vi "项操作.vi"(8 "error in (no error)":errorcluster caption="错误输入（无错误）", 9 "Cell Position":T1, 10 "MCListbox引用句柄":refnum<vi>, 11 "LNK 输入":refnum<class "Hide Row.lvclass">) -> (0 "error out":errorcluster caption="错误输出", 3 "LNK 输出":refnum<class "Hide Row.lvclass">)   [LabVIEW 2016, in "Hide Row.lvclass"]
uses:
  Hide Row.lvclass
  <vilib>/Utility/miscctls.llb/LVRowAndColumnTypeDef.ctl
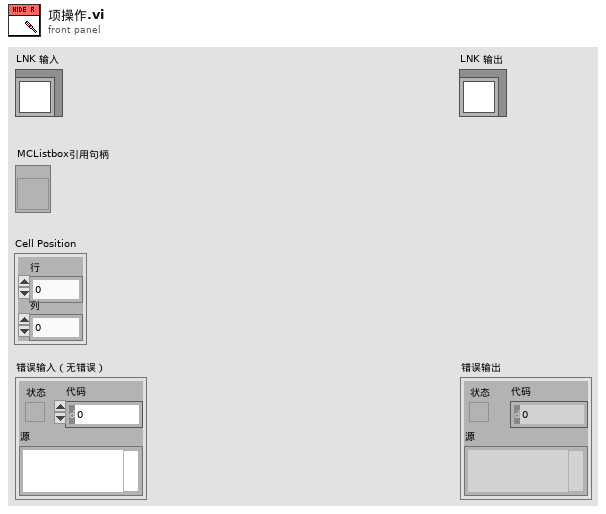
[diagram p1: front panel]
types:
  T1 = typedef "LVRowAndColumnTypeDef.ctl" = cluster{"Row":i32, "Column":i32}
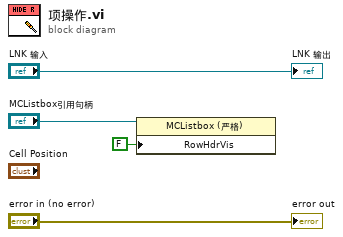
[diagram p0: block diagram]
diagram:
  n1 = property class="MCListbox (严格)"(reference="MCListbox引用句柄", "RowHdrVis"=FALSE ("显示项:显示行首")) -> ()  [unwired: 1 in, 2 out]
  "error out" <- "error in (no error)"
  "LNK 输出" <- "LNK 输入"
